vi "MathOptim-Logistic Model.vi"(3 "output control":T1, 4 "data":variant, 5 "X":dbl[](array[numeric]), 6 "a":dbl[](array[numeric])) -> (0 "error out":errorcluster, 1 "f'(X,a)":dbl[][](array[numeric]), 2 "f(X,a)":dbl[](array[numeric]))   [LabVIEW 2015]
doc: "This template is the starting point for creating a model function to be passed to the Nonlinear Curve Fit.vi."
uses:
  <vilib>/gmath/NumericalOptimization/LM_output select.ctl
  <vilib>/Analysis/7linalg.llb/Solve Linear Equations (single right hand).vi
  <vilib>/Analysis/baseanly.llb/Solve Linear Equations By Cholesky.vi
  <vilib>/Analysis/baseanly.llb/Real Matrix to Compact Array.vi
  <vilib>/Analysis/baseanly.llb/Real Compact Tri-Matrix Linear Eqs.vi
  <vilib>/Analysis/7linalg.llb/Solve Linear Eqs (General).vi
  <vilib>/Analysis/7linalg.llb/Solve Linear Eqs (Gen, single right hand).vi
  <vilib>/Analysis/NI_AALPro.lvlib
  <vilib>/gmath/NI_Gmath.lvlib
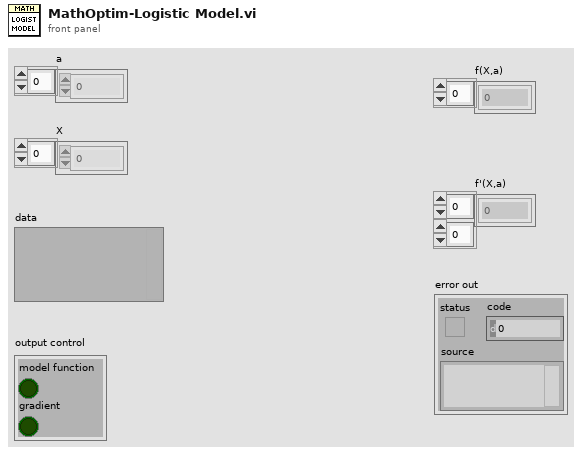
[diagram p1: front panel]
types:
  T1 = typedef "NI_Gmath.lvlib/LM_output select.ctl" = cluster{"model function":bool, "gradient":bool}
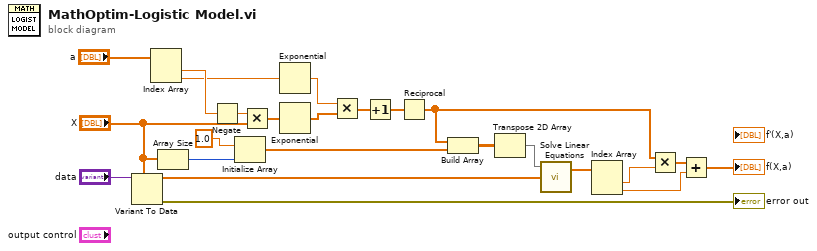
[diagram p0: block diagram]
diagram:
  n1 = Variant To Data(type="X", Variant="data") -> (data=w21:dbl[], error out=→"error out":errorcluster)  [unwired: 1 in]
  n2 = Index Array(array="a") -> (element #1=w9:dbl, element #2=w7:dbl)  [unwired: 2 in]
  n3 = Array Size(array="X") -> (size(s)=w20:i32)
  n4 = Negate(x=w9) -> (-x=w1:dbl)
  n5 = Initialize Array(1.0, w20) -> (w18:dbl[])
  n6 = Multiply(x=w1, y="X") -> (x*y=w8:dbl[])
  n7 = Exponential(1:w7) -> (0:w6:dbl)
  n8 = Exponential(1:w8) -> (0:w5:dbl[])
  n9 = Multiply(x=w6, y=w5) -> (x*y=w4:dbl[])
  n10 = Increment(x=w4) -> (x+1=w3:dbl[])
  n11 = Reciprocal(x=w3) -> (1/x=w2:dbl[])
  n12 = Build Array(w2, w18) -> (w17:dbl[][])
  n13 = Transpose 2D Array(2D array=w17) -> (transposed array=w11:dbl[][])
  n14 = call-poly <vilib>:"Solve Linear Equations.vi"("Known Vector"=w21, "Input Matrix"=w11) -> ("Solution Vector"=w16:dbl[])  [unwired: 1 in, 1 out]
  n15 = Index Array(array=w16) -> (element #1=w15:dbl, element #2=w13:dbl)  [unwired: 2 in]
  n16 = Multiply(x=w2, y=w15) -> (x*y=w14:dbl[])
  n17 = Add(x=w14, y=w13) -> (x+y=→"f(X,a)":dbl[])
